vi "WPI_DigitalModuleGetPWM.vi"(8 "error in (no error)":errorcluster, 10 "PWMChannel":T1, 11 "DigitalModuleDevRef":T2) -> (0 "error out":errorcluster, 2 "Speed":u16, 3 "DigitalModuleDevRef":T2)   [LabVIEW 2017]
doc: "This software is licensed. Open the labview\\readme\\WPI Robotics Library Open Source License.txt file for more information."
uses:
  <vilib>/Rock Robotics/WPI/DigitalModule/WPI_DigitalModuleDeviceRef.ctl
  <vilib>/Rock Robotics/SystemInterfaces/DIO/FPGA_DIOPWMChannel.ctl
  <vilib>/Rock Robotics/SystemInterfaces/System/FPGA_SystemGet.vi
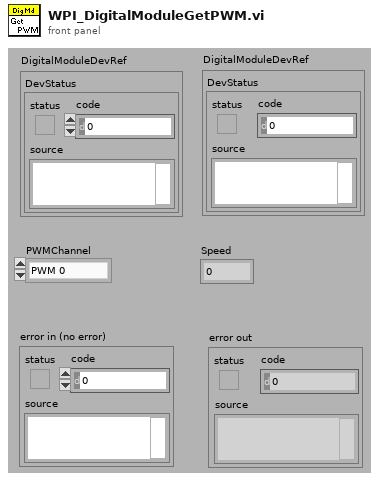
[diagram p1: front panel]
types:
  T1 = typedef "FPGA_DIOPWMChannel.ctl" = enum8{"PWM 0", "PWM 1", "PWM 2", "PWM 3", "PWM 4", "PWM 5", "PWM 6", "PWM 7", "PWM 8", "PWM 9", "PWM MXP 0", "PWM MXP 1", "PWM MXP 2", "PWM MXP 3", "PWM MXP 4", "PWM MXP 5", "PWM MXP 6", "PWM MXP 7", "PWM MXP 8", "PWM MXP 9", "Invalid"}
  T2 = typedef "WPI_DigitalModuleDeviceRef.ctl" = cluster{"DevStatus":errorcluster}
  T3 = typedef "FPGA_DIODevRef.ctl" = cluster{"DevStatus":errorcluster}
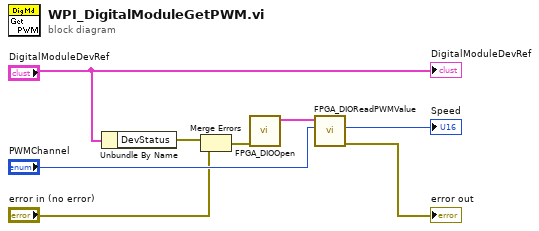
[diagram p0: block diagram]
diagram:
  n1 = Unbundle By Name("DigitalModuleDevRef") -> ("DevStatus"=w4:errorcluster)
  n2 = Merge Errors(w4, "error in (no error)") -> (w3:errorcluster)
  n3 = call <vilib>:"FPGA_DIOOpen.vi"("error in (no error)"=w3) -> ("DIODeviceRef"=w5:T3)  [unwired: 1 in, 9 out]
  n4 = call <vilib>:"FPGA_DIOReadPWMValue.vi"("PWMChannel"="PWMChannel", "DIODeviceRef In"=w5) -> ("error out"=→"error out":errorcluster, "PWMValue"=→"Speed":u16)  [unwired: 1 in, 7 out]
  "DigitalModuleDevRef" <- "DigitalModuleDevRef"
